vi "Lookup Table Generator.vi"() -> ()   [LabVIEW 2013]
uses:
  <vilib>/Math Plots/2D Math Plots/2D Compass/2D Compass XCtrl/2D Compass.xctl
  Reference Global.vi
panel:
  out "Within\nBoundary":bool
  out "Y Max":dbl
  out "X of Y max":dbl
  out "Lookup Table":string[][](table)
  in  "Speed (rpm)":dbl
  out "Table":string[][](table)
  in  "Delta Time":dbl
  out "Y Coordinate Initial distance from ultrasonic":dbl
  out "X Coordinate Initial distance from ultrasonic":dbl
  out "Initial Throw Angle Graph":refnum<class "2D Plot Datatype.lvclass">[](xcontrol) caption="2D Compass"
  out "Angle of Catapult":dbl
  out "Angle of Throw":dbl
  out "Initial Y Delta (m)":dbl
  out "Initial X Delta (m)":dbl
  out "Angle of Throw Relative to Forward Horizantal = 0":dbl
  out "Angular Velocity":dbl
  in  "Catapult Move\nAngle":dbl
  # "0.01 is optimal"
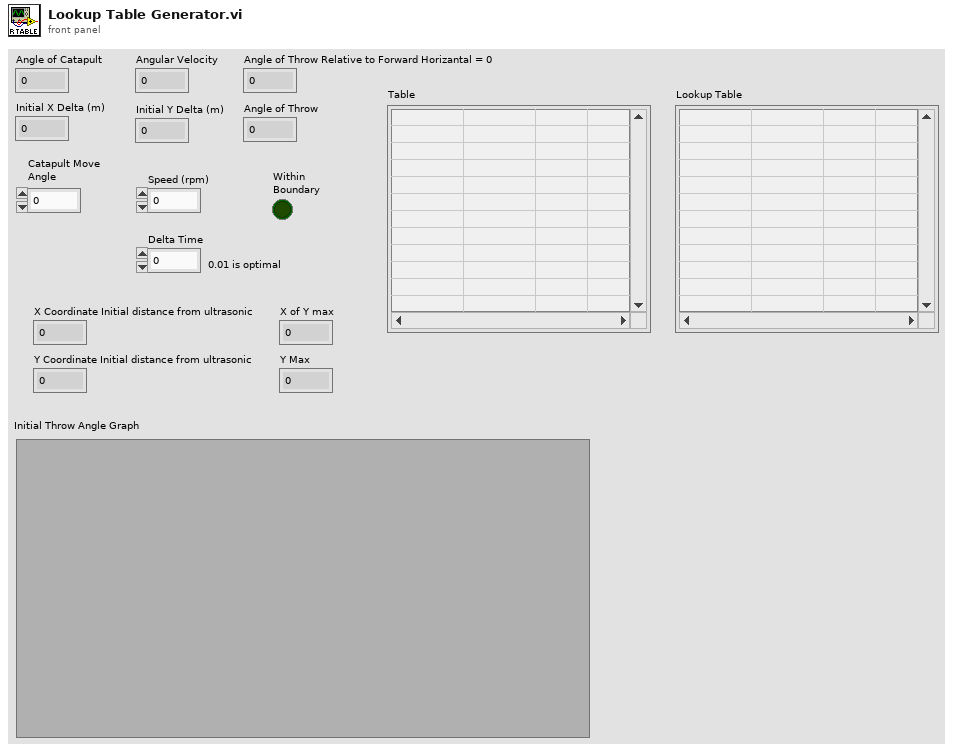
[diagram p1: front panel]
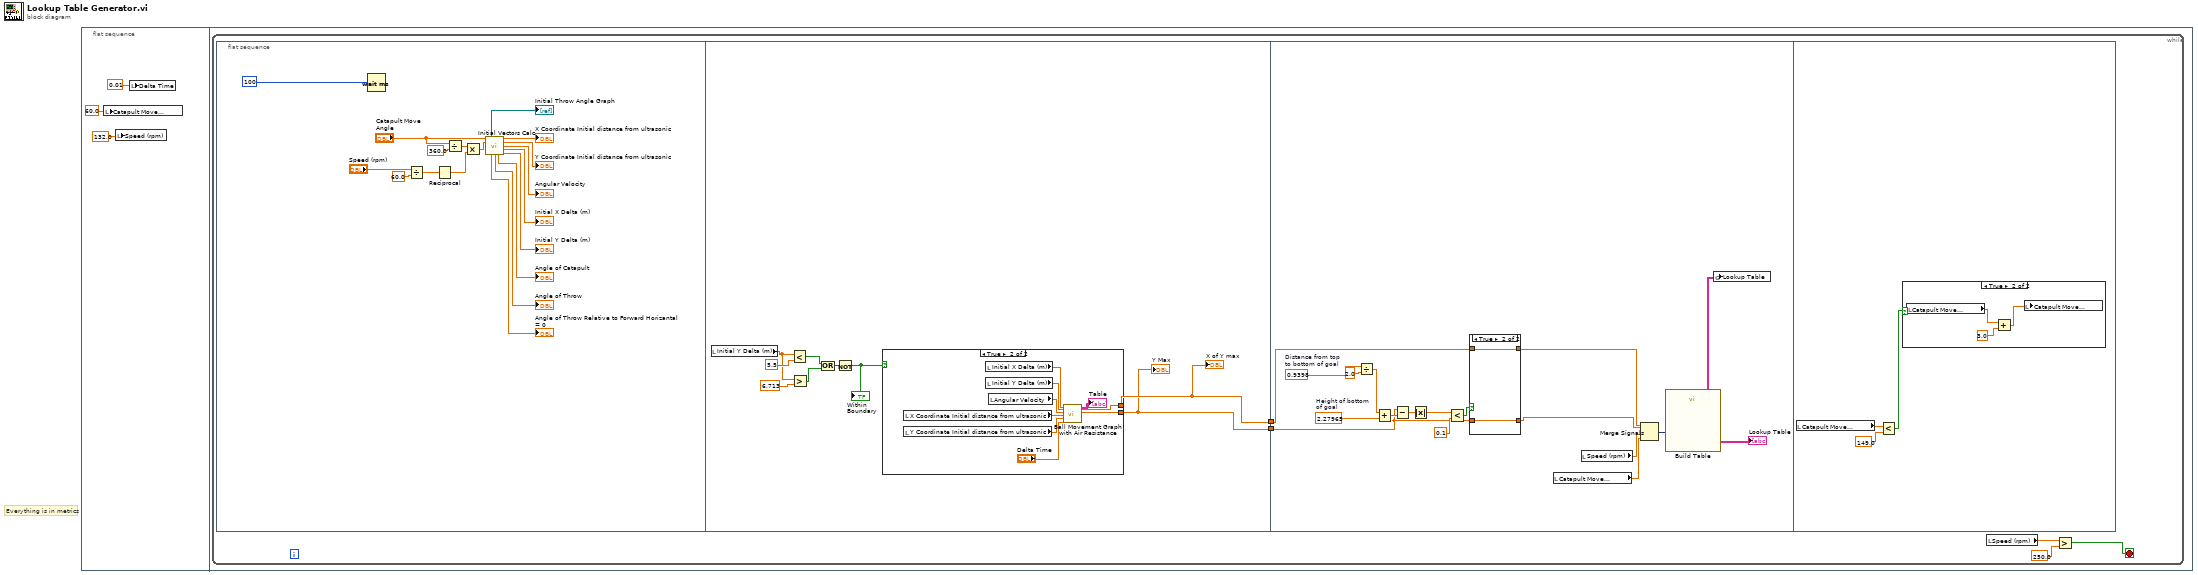
[diagram p0: block diagram]
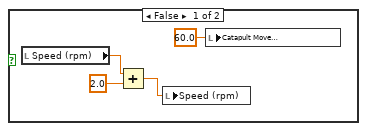
[diagram p4: hidden frame]
diagram:
  # "Everything is in metrics"
  n1 = flat-sequence {
    frame #0 {
      n2 = local write "Catapult Move\nAngle"(60.0 ("Catapult Move\nAngle")) -> ()
      n3 = local write "Speed (rpm)"(132.0 ("Speed (rpm)")) -> ()
      n4 = local write "Delta Time"(0.01 ("Delta Time")) -> ()
    }
    frame #1 {
      n5 = while {
        stop <- w6 stop-if-true
        n6 = flat-sequence {
          tunnel: [w35] -> w5
          tunnel: [w34] -> w4
          tunnel: w5 -> [w51]
          tunnel: w4 -> [w52]
          frame #0 {
            n7 = Wait (ms)(milliseconds to wait=u32 100) -> ()  [unwired: 1 out]
            n8 = Divide(x="Speed (rpm)", y=60.0) -> (x/y=w21:dbl)
            n9 = Reciprocal(x=w21) -> (1/x=w24:dbl)
            n10 = Divide(x="Catapult Move\nAngle", y=360.0) -> (x/y=w23:dbl)
            n11 = Multiply(x=w23, y=w24) -> (x*y=w20:dbl)
            n12 = call "Initial Vectors Calc.vi"("Catapult Move\nAngle"="Catapult Move\nAngle", "Time of Rotation"=w20) -> ("2D Plot Class Obj Array out"=→"Initial Throw Angle Graph":refnum<class "2D Plot Datatype.lvclass">[], "X Initial distance from ultrasonic"=→"X Coordinate Initial distance from ultrasonic":dbl, "Y Initial distance from ultrasonic"=→"Y Coordinate Initial distance from ultrasonic":dbl, "Angular Velocity"=→"Angular Velocity":dbl, "X Delta (m)"=→"Initial X Delta (m)":dbl, "Angle of Throw Relative to Forward Horizantal = 0"=→"Angle of Throw Relative to Forward Horizantal = 0":dbl, "Angle of Throw"=→"Angle of Throw":dbl, "Angle of Catapult"=→"Angle of Catapult":dbl, "Y Delta (m)"=→"Initial Y Delta (m)":dbl)  [unwired: 5 in]
          }
          frame #1 {
            n13 = local read "Initial Y Delta (m)"() -> (w27:dbl)
            n14 = Less?(x=w27, y=5.5) -> (x < y?=w31:bool)
            n15 = Greater?(x=w27, y=6.713) -> (0:w30:bool)
            n16 = Or(x=w31, y=w30) -> (x .or. y?=w29:bool)
            n17 = Not(x=w29) -> (.not. x?=w28:bool)
            "Within\nBoundary" <- w28
            n18 = case shown="True" w28 {
              tunnel: [_ w39] -> w35
              tunnel: [_ w38] -> w34
              frame False {
              }
              frame True {
                n19 = local read "X Coordinate Initial distance from ultrasonic"() -> (w37:dbl)
                n20 = local read "Y Coordinate Initial distance from ultrasonic"() -> (w36:dbl)
                n21 = local read "Initial X Delta (m)"() -> (w42:dbl)
                n22 = local read "Initial Y Delta (m)"() -> (w41:dbl)
                n23 = local read "Angular Velocity"() -> (w43:dbl)
                n24 = call "Ball Movement Graph with Air Resistance.vi"("X Velocity Initial"=w42, "Y Velocity Initial"=w41, "Initial Angular Velocity"=w43, "X Coordinate Initial"=w37, "Y Coordinate Initial"=w36, "Delta Time"="Delta Time") -> ("Table"=→"Table":string[][], "X of Y max"=w39:dbl, "Y Max"=w38:dbl)  [unwired: 9 in, 2 out]
              }
            }
            "X of Y max" <- w35
            "Y Max" <- w34
          }
          frame #2 {
            w58 = 2.27965  # Height of bottom  of goal
            w60 = 0.9398  # Distance from top to bottom of goal
            n25 = Divide(x=w60, y=2.0) -> (x/y=w59:dbl)
            n26 = Add(x=w59, y=w58) -> (x+y=w57:dbl)
            n27 = Subtract(x=w52, y=w57) -> (x-y=w56:dbl)
            n28 = Absolute Value(x=w56) -> (abs(x)=w55:dbl)
            n29 = Less?(x=w55, y=0.1) -> (x < y?=w53:bool)
            n30 = case shown="True" w53 {
              tunnel: w52 -> [_ w62]
              tunnel: w51 -> [_ w63]
              tunnel: [_ w63] -> w50
              tunnel: [_ w62] -> w46
              frame False {
              }
              frame True {
              }
            }
            n31 = local read "Catapult Move\nAngle"() -> (w48:dbl)
            n32 = local read "Speed (rpm)"() -> (w49:dbl)
            n33 = Merge Signals(w50, w46, w49, w48) -> (w47:dynamicdata)
            n34 = call "Build Table"("Signals"=w47) -> ("Table"=w45:string[][])  [unwired: 4 in, 6 out]
            "Lookup Table" <- w45
            n35 = global write "Reference Global.vi" "Lookup Table"(w45) -> ()
          }
          frame #3 {
            n36 = local read "Catapult Move\nAngle"() -> (w66:dbl)
            n37 = Less?(x=w66, y=149.0) -> (x < y?=w64:bool)
            n38 = case shown="True" w64 {
              frame False {
                n39 = local read "Speed (rpm)"() -> (w69:dbl)
                n40 = Add(x=w69, y=2.0) -> (x+y=w68:dbl)
                n41 = local write "Speed (rpm)"(w68) -> ()
                n42 = local write "Catapult Move\nAngle"(60.0 ("Catapult Move\nAngle")) -> ()
              }
              frame True {
                n43 = local read "Catapult Move\nAngle"() -> (w72:dbl)
                n44 = Add(x=w72, y=3.0) -> (x+y=w73:dbl)
                n45 = local write "Catapult Move\nAngle"(w73) -> ()
              }
            }
          }
        }
        n46 = local read "Speed (rpm)"() -> (w7:dbl)
        n47 = Greater?(x=w7, y=250.0) -> (0:w6:bool)
      }
    }
  }
